vi "main.vi"() -> ()   [LabVIEW 2010]
uses:
  <vilib>/Platform/TimedLoop/XDataNode/wakeup.ctl
  <vilib>/Platform/TimedLoop/XDataNode/XDNodeRunTimeDep.lvlib
  <vilib>/Platform/TimedLoop/XDataNode/nitl_modes.ctl
  <vilib>/Platform/TimedLoop/XDataNode/timing_clust.ctl
  <vilib>/Platform/TimedLoop/XDataNode/XDataNode.xnode
  <vilib>/rvi/DataTransferAndStorage/Container/XNode/niFpgaContainer.xnode
  <vilib>/eio/EIONode/EIONode.xnode
  FPGA VIs/counter_cluster_flexRIO.ctl
  FPGA VIs/integration_cluster_flexRIO.ctl
  <vilib>/rvi/eio/nirviEIOImplementation/nirviEIOImplementation.xnode
  <vilib>/rvi/eio/common/nirviEmuTemplateMethod_noerrors.vi
  <vilib>/rvi/eio/common/nirviEmuClasses.ctl
  <vilib>/rvi/FIFO/Fifo_Resource/nirvififoEmulationSetSize.vi
  <vilib>/rvi/DataTransferAndStorage/Container/Common/niFpgaContainerGetUniqueNameForEmu.vi
  FPGA VIs/OnBoardBuffer_flexRIO Folder/OnBoardBuffer_flexRIO.lvlib
  FPGA VIs/OnBoardBuffer_flexRIO Folder/OnBoardBuffer_flexRIO.ctl
  common_typedefs/gate_parameters_cluster.ctl
  FPGA VIs/scan_specification_cluster_flexRIO.ctl
  FPGA VIs/derived_values_cluster_flexRIO.ctl
  FPGA VIs/DAC_voltage_cluster_flexRIO.ctl
  FPGA VIs/channels_cluster_flexRIO.ctl
  FPGA VIs/write_to_fifo_status_flexRIO.ctl
panel:
  out "read output":T1
  in  "channel offsets":T1
  out "derived values":T2
  out "integration loop counter":i32
  out "transferred z/intensity tuples":u32
  out "no of correct transferred z tuples":u32
  out "z-points transfer corrupt?":bool
  in  "transfer z-points?":bool
  out "transferred extra waitlines":u32
  in  "transfer extra-waitlines?":bool
  out "counter cluster out":T3
  out "pixels acquired":u64
  in  "scan":bool
  in  "wait for trigger?":bool
  in  "stop acquisition at\nFIFO overflow?":bool
  out "scanning?":bool
  out "loop-to-loop FIFO overflow":bool
  in  "stop":bool
  in  "scan specification":T4={"x amplitude"=1000, "x resolution (pixels)"=200, "x offset fly-forward (iterations)"=0, "x offset fly-back (iterations)"=0, "y resolution (nr. of lines)"=200, "y step size"=5, "iterations per pixel"=5, "number of frames"=-1, "y offset (pixels)"=0, "number of y-brake lines  (before y-fly-back)"=2, "number y-brake lines (after y-fly-back)"=2, "number of y-fly-back steps"=2, "lines per z step"=0, "number of z/intensity tuples"=0, "number of repetitions (volumes or planes)"=0}
  out "DAC voltages":T5 {"ch6" max=4095 step=1; "ch5" max=4095 step=1; "ch4" max=4095 step=1; "ch3" max=4095 step=1; "ch2" max=4095 step=1; "ch1" max=4095 step=1; "ch0" max=4095 step=1}
  out "acquire?":bool
  in  "sync minimum high":i16=1000
  in  "maximum bit depth":i8
  in  "enable fly-back reversion?":bool=TRUE
  in  "invert channels":bool[](array[boolean])=[FALSE, FALSE]
  out "no. elements in on-board buffer":u32
  out "on-board buffer":T6
  out "target-to-host FIFO full?":bool
  out "write-to-FIFO status":T7
  out "data received for buffering":u32
  in  "clock 1":T8
  in  "clock 2":T8
  in  "clock 3":T8
  out "clock 2 state":bool
  out "clock 1 state":bool
  out "clock 3 state":bool
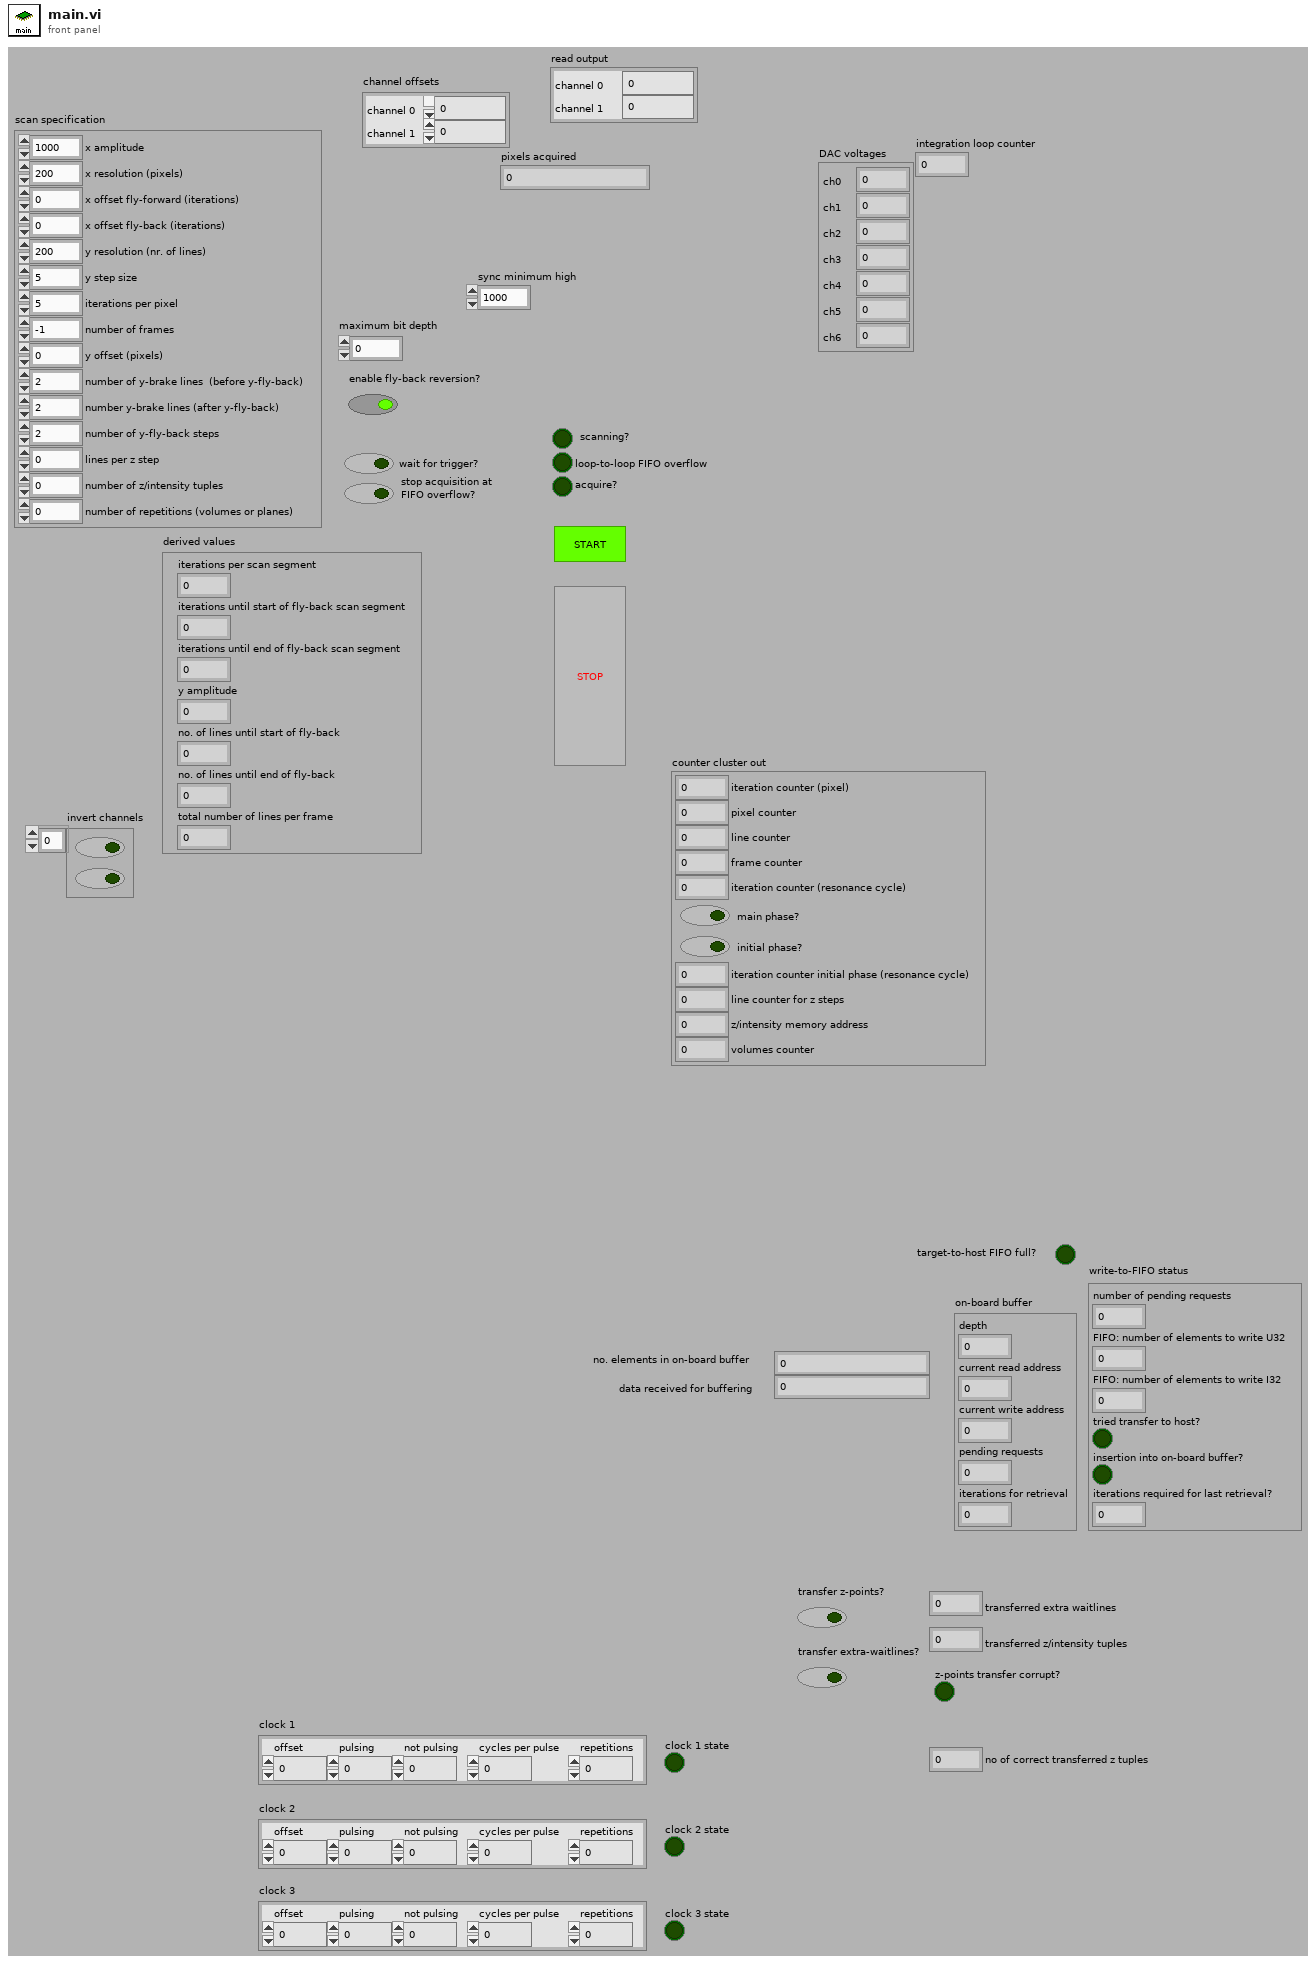
[diagram p1: front panel]
types:
  T1 = typedef "channels_cluster_flexRIO.ctl" = cluster{"channel 0":u32, "channel 1":u32}
  T2 = typedef "derived_values_cluster_flexRIO.ctl" = cluster{"iterations per scan segment":u16, "iterations until start of fly-back scan segment":u16, "iterations until end of fly-back scan segment":u16, "y amplitude":u16, "no. of lines until start of fly-back":u16, "no. of lines until end of fly-back":u16, "total number of lines per frame ":u16}
  T3 = typedef "counter_cluster_flexRIO.ctl" = cluster{"iteration counter (pixel)":u16, "pixel counter":u16, "line counter":u16, "frame counter":u16, "iteration counter (resonance cycle)":u16, "main phase?":bool, "initial phase?":bool, "iteration counter initial phase (resonance cycle)":u16, "line counter for z steps":u16, "z/intensity memory address":u32, "volumes counter":u16}
  T4 = typedef "scan_specification_cluster_flexRIO.ctl" = cluster{"x amplitude":u16, "x resolution (pixels)":u16, "x offset fly-forward (iterations)":u16, "x offset fly-back (iterations)":u16, "y resolution (nr. of lines)":u16, "y step size":u16, "iterations per pixel":u16, "number of frames":i32, "y offset (pixels)":u16, "number of y-brake lines  (before y-fly-back)":u16, "number y-brake lines (after y-fly-back)":u16, "number of y-fly-back steps":u16, "lines per z step":u16, "number of z/intensity tuples":u16, "number of repetitions (volumes or planes)":i32}
  T5 = typedef "DAC_voltage_cluster_flexRIO.ctl" = cluster{"ch0":u16, "ch1":u16, "ch2":u16, "ch3":u16, "ch4":u16, "ch5":u16, "ch6":u16}
  T6 = typedef "OnBoardBuffer_flexRIO.lvlib/OnBoardBuffer_flexRIO.ctl" = cluster{"depth":u32, "current read address":u32, "current write address":u32, "pending requests":u32, "iterations for retrieval":u32}
  T7 = typedef "write_to_fifo_status_flexRIO.ctl" = cluster{"number of pending requests":i32, "FIFO: number of elements to write U32":u32, "FIFO: number of elements to write I32":i32, "tried transfer to host?":bool, "insertion into on-board buffer?":bool, "iterations required for last retrieval?":u32}
  T8 = typedef "gate_parameters_cluster.ctl" = cluster{"offset":i64, "pulsing":i64, "not pulsing":i64, "cycles per pulse":i64, "repetitions":i64}
  T9 = typedef "integration_cluster_flexRIO.ctl" = cluster{"channel 0":u32, "channel 1":u32, "fly-back heap address":u32}
  T10 = typedef "XDNodeRunTimeDep.lvlib/timing_clust.ctl" = cluster{"Expected End [f-1]":u64, "Actual End [f-1]":u64, "Finished Late? [f-1]":bool, "Expected End [i-1]":u64, "Actual End [i-1]":u64, "Finished Late? [i-1]":bool, "Expected Start [i]":u64, "Actual Start [i]":u64, "Expected Start [f]":u64, "Actual Start [f]":u64, "Source Name":string, "Structure Name":string, "Period":i64, "Deadline":i64, "Offset":i64, "Start":i64, "Priority":i32, "Timeout":i32, "Mode":T11, "Wakeup Reason":T12, "Error":errorcluster, "Source Type":string, "Secondary Source Type":string, "Global End Time":u64, "Global Start Time":u64, "Frame Duration":u64, "Iteration Duration":u64, "Assigned CPU":i32, "I/O Scan Engine Mode":u32}
  T11 = typedef "XDNodeRunTimeDep.lvlib/nitl_modes.ctl" = enum32{"No Change", "Process missed periods, maintain original phase", "Discard missed periods, maintain original phase", "Process missed periods, ignore original phase", "Discard missed periods, ignore original phase"}
  T12 = typedef "XDNodeRunTimeDep.lvlib/wakeup.ctl" = enum32{"Normal", "Aborted", "Asynchronous wakeup", "Timing source error", "Timed loop error", "Timeout"}
  T13 = typedef "nirviEmuClasses.ctl" = enum16{"IO Read", "IO Write", "Method", "Property Read", "Property Write"}
  T14 = typedef "gate_counters_cluster.ctl" = cluster{"phase iteration counter":i64, "phase repetition counter":i64, "pulse iteration counter":i64, "phase state":bool}
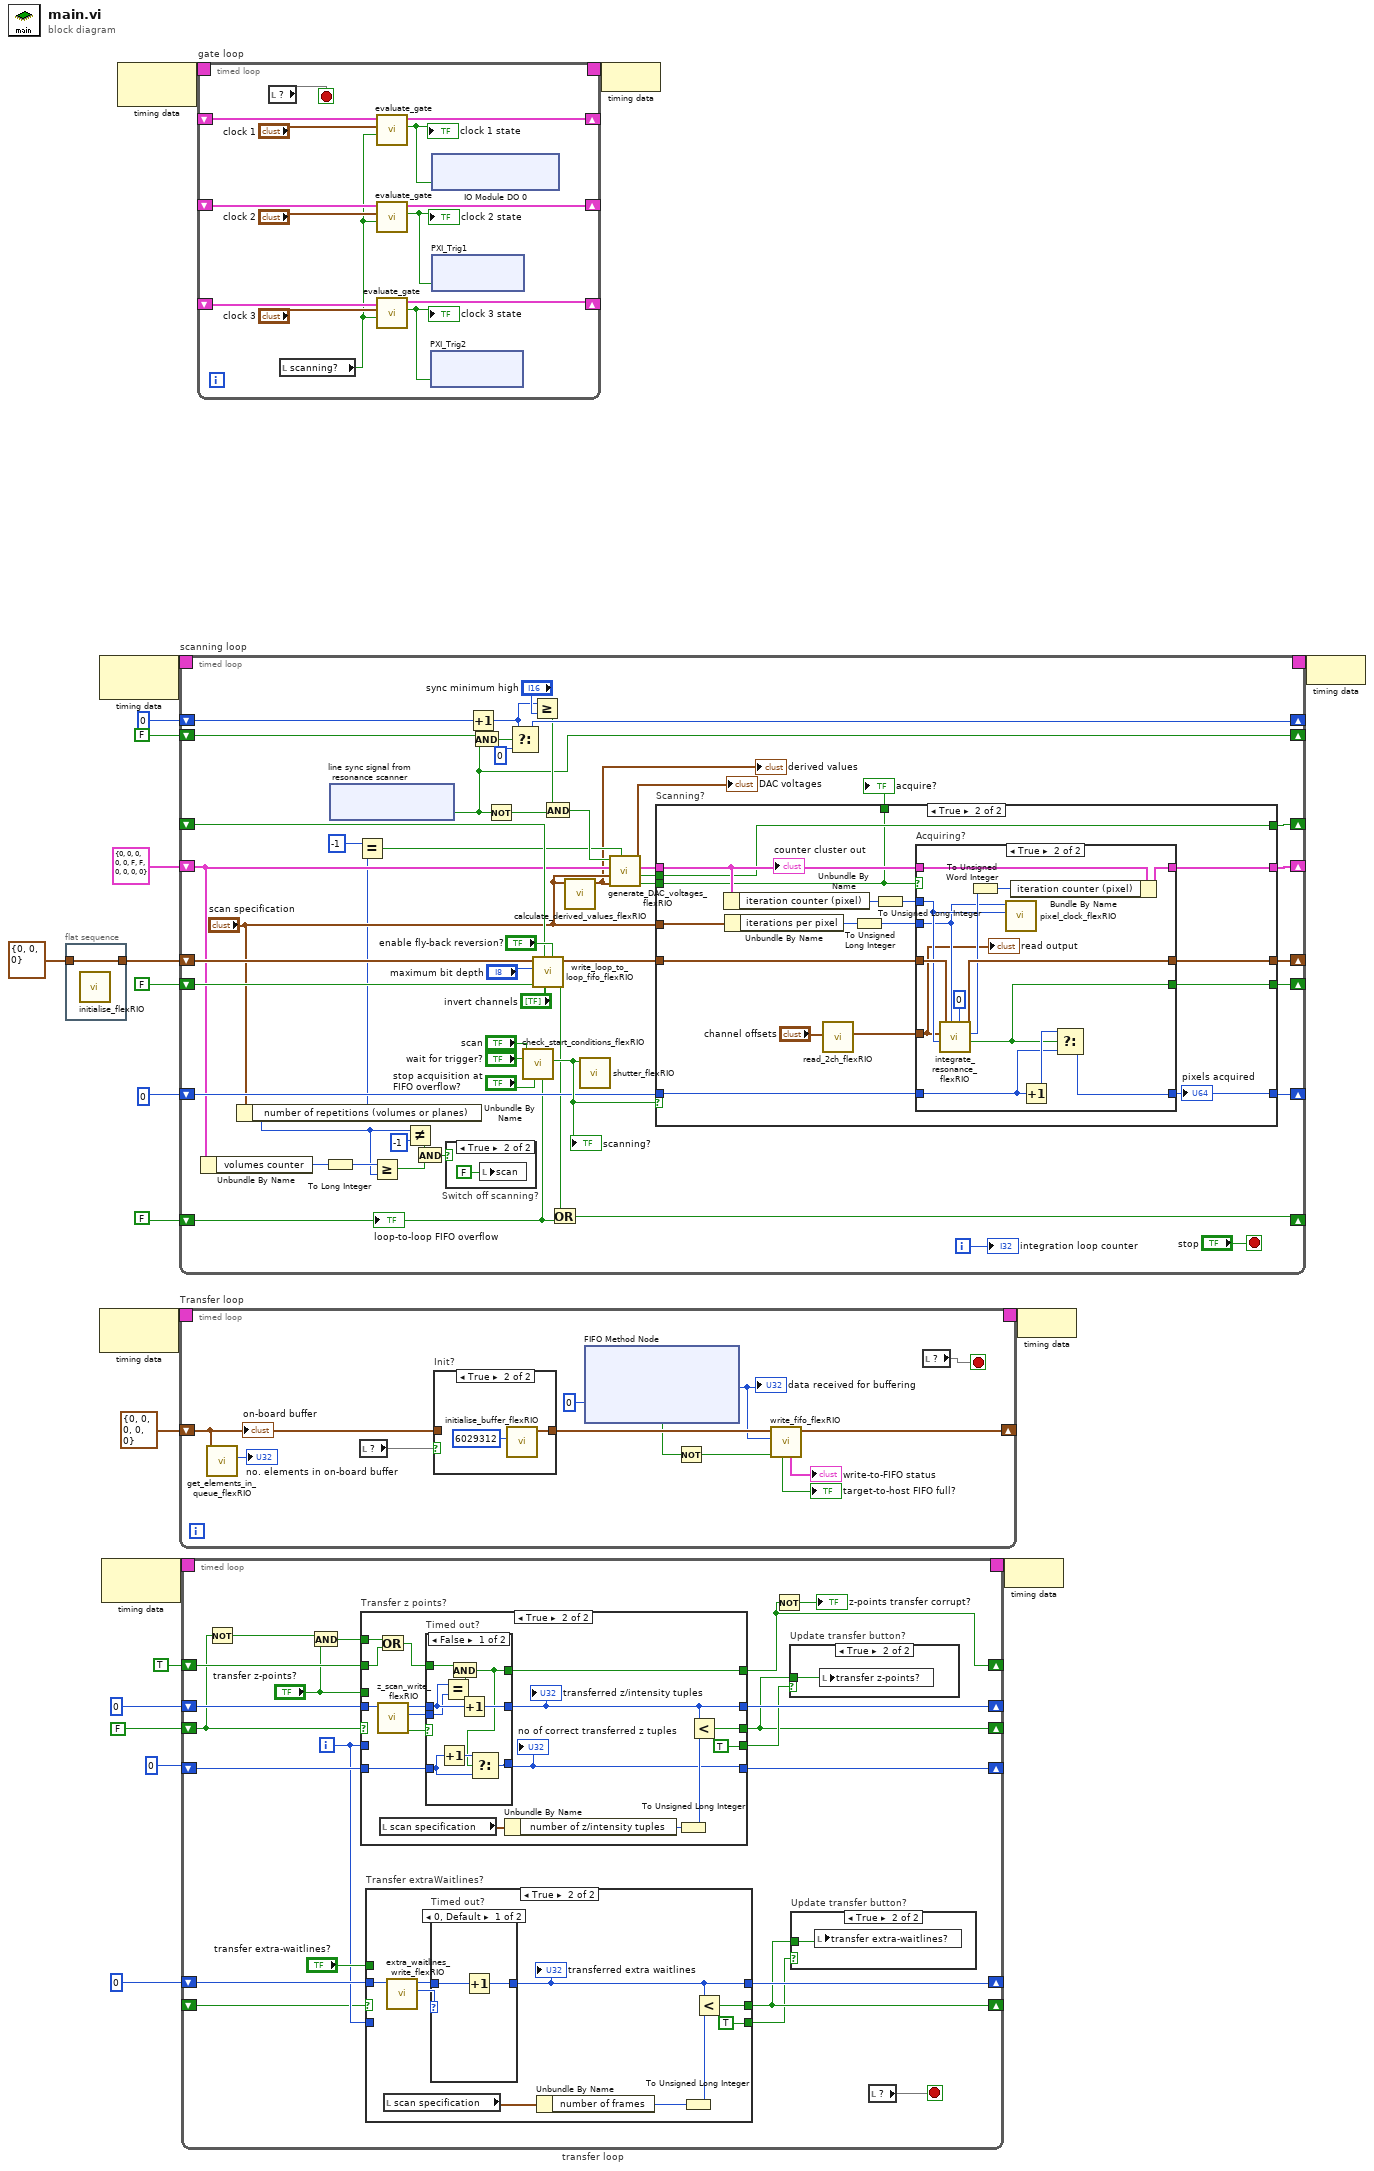
[diagram p0: block diagram]
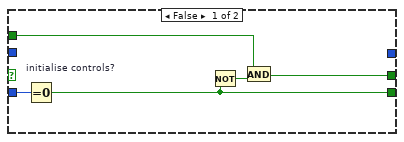
[diagram p3: hidden frame]
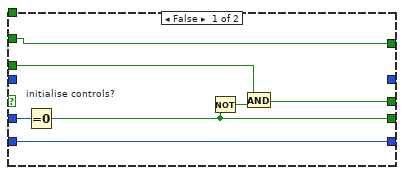
[diagram p6: hidden frame]
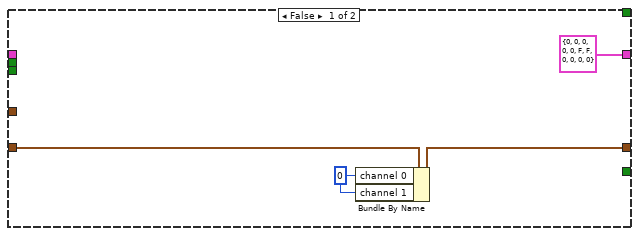
[diagram p9: hidden frame]
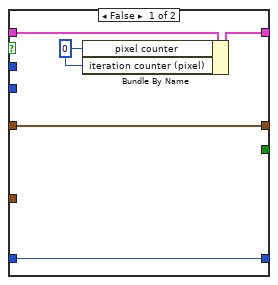
[diagram p10: hidden frame]
diagram:
  n1 = flat-sequence {
    tunnel: T9 {"channel 0"=0, "channel 1"=0, "fly-back heap address"=0} ("integration cluster") -> [w23]
    tunnel: [w23] -> w2
    frame #0 {
      n2 = call "initialise_flexRIO.vi"() -> ()  [unwired: 12 in]
    }
  }
  n3 = node-c288() -> (w18:T10)  [unwired: 1 in]
  n4 = node-c288() -> (w20:T10)  [unwired: 1 in]
  n5 = node-c288() -> (w10:T10)  [unwired: 1 in]
  n6 = node-c288() -> (w22:T10)  [unwired: 1 in]
  n7 = timed-loop "scanning loop" {
    timing: w18 -> [_]
    timing-out: [_] -> w17
    shift-right: [w71] -> _
    shift-left: T3 {"iteration counter (pixel)"=0, "pixel counter"=0, "line counter"=0, "frame counter"=0, "iteration counter (resonance cycle)"=0, "main phase?"=FALSE, "initial phase?"=FALSE, "iteration counter initial phase (resonance cycle)"=0, "line counter for z steps"=0, "z/intensity memory address"=0, "volumes counter"=0} ("counter cluster") -> [w37]
    shift-right: [w48] -> _
    shift-left: w2 -> [w47]
    shift-right: [w26] -> _
    shift-left: FALSE -> [w41]
    shift-right: [w40] -> _
    shift-left: FALSE -> [w60]
    shift-right: [w62] -> _
    shift-left: u64 0 -> [w63]
    shift-right: [w56] -> _
    shift-left: i16 0 -> [w59]
    shift-right: [w49] -> _
    shift-left: _ -> [w45]
    shift-right: [w43] -> _
    shift-left: FALSE ("finished?") -> [w42]
    i -> [w25]
    stop <- "stop" stop-if-true
    n8 = Unbundle By Name(w37) -> ("volumes counter"=w31:u16)
    n9 = Unbundle By Name("scan specification") -> ("number of repetitions (volumes or planes)"=w29:i32)
    n10 = To Long Integer(number=w31) -> (32bit integer=w30:i32)
    n11 = xnode "line sync signal from\nresonance scanner"() -> ("IO Module\\DI 1"=w40:bool)  [unwired: 1 in, 1 out]
    n12 = Equal?(x=-1, y=w29) -> (x = y?=w27:bool)
    n13 = Greater Or Equal?(x=w30, y=w29) -> (x >= y?=w68:bool)
    n14 = Not Equal?(x=w29, y=-1) -> (x != y?=w65:bool)
    n15 = And(x=w65, y=w68) -> (x .and. y?=w64:bool)
    n16 = case "Switch off scanning?" shown="True" w64 {
      frame False {
      }
      frame True {
        n17 = local write "scan"(FALSE ("scan")) -> ()
      }
    }
    n18 = Increment(x=w59) -> (x+1=w54:i16)
    n19 = And(x=w60, y=w40) -> (x .and. y?=w58:bool)
    n20 = Not(x=w40) -> (.not. x?=w53:bool)
    n21 = Select(t=w54, s=w58, f=i16 0) -> (s? t:f=w56:i16)
    n22 = call "check_start_conditions_flexRIO.vi"("FIFO overflow?"=w41, "stop at FIFO overflow?"="stop acquisition at\nFIFO overflow?", "in triggered mode?"="wait for trigger?", "acquire"="scan") -> ("acquire?"=w66:bool)  [unwired: 7 in]
    "scanning?" <- w66
    n23 = Greater Or Equal?(x=w54, y="sync minimum high") -> (x >= y?=w52:bool)
    n24 = call "write_loop_to_loop_fifo_flexRIO.vi"("enable fly-back reversion?"="enable fly-back reversion?", "invert channels"="invert channels", "fly-back?"=w45, "pixel finished?"=w42, "maximum bit depth"="maximum bit depth", "integration cluster in"=w47) -> ("local transfer FIFO full"=w44:bool, "integration cluster out"=w46:T9)  [unwired: 4 in]
    n25 = And(x=w52, y=w53) -> (x .and. y?=w38:bool)
    n26 = Or(x=w44, y=w41) -> (x .or. y?=w26:bool)
    n27 = call "calculate_derived_values_flexRIO.vi"("scan specification"="scan specification") -> ("derived values"=w24:T2)  [unwired: 10 in]
    "derived values" <- w24
    n28 = call "shutter_flexRIO.vi"("open?"=w66) -> ()  [unwired: 11 in]
    n29 = call "generate_DAC_voltages_flexRIO.vi"("focus mode?"=w27, "derived values"=w24, "scan specification"="scan specification", "counter cluster in"=w37, "resonant trigger"=w38) -> ("acquire?"=w33:bool, "fly-back acquisition phase?"=w34:bool, "counter cluster out"=w36:T3, "DAC voltages"=→"DAC voltages":T5)  [unwired: 3 in]
    n30 = case "Scanning?" shown="True" w66 {
      tunnel: w36 -> [_ w101]
      tunnel: [T3 {"iteration counter (pixel)"=0, "pixel counter"=0, "line counter"=0, "frame counter"=0, "iteration counter (resonance cycle)"=0, "main phase?"=FALSE, "initial phase?"=FALSE, "iteration counter initial phase (resonance cycle)"=0, "line counter for z steps"=0, "z/intensity memory address"=0, "volumes counter"=0} ("counter cluster") w113] -> w71
      tunnel: w46 -> [w95 w109]
      tunnel: [w94 w112] -> w48
      tunnel: "scan specification" -> [_ w102]
      tunnel: w63 -> [_ w105]
      tunnel: [_ w104] -> w62
      tunnel: [_ w99] -> w61
      tunnel: [_ w103] -> w43
      tunnel: [_ w100] -> w49
      tunnel: w34 -> [_ w100]
      tunnel: w33 -> [_ w99]
      frame False {
        w96 = u32 0 ("channel 0")
        n31 = Bundle By Name(cluster=w95, "channel 0"=w96, "channel 1"=w96) -> (w94:T9)
      }
      frame True {
        n32 = Unbundle By Name(w101) -> ("iteration counter (pixel)"=w111:u16)
        n33 = Unbundle By Name(w102) -> ("iterations per pixel"=w110:u16)
        n34 = call "read_2ch_flexRIO.vi"("channel offsets"="channel offsets") -> ("read output"=w107:T1)  [unwired: 10 in]
        n35 = To Unsigned Long Integer(number=w110) -> (unsigned 32bit integer=w106:u32)
        n36 = To Unsigned Long Integer(number=w111) -> (unsigned 32bit integer=w108:u32)
        n37 = case "Acquiring?" shown="True" w99 {
          tunnel: w101 -> [w117 w129]
          tunnel: [w118 w128] -> w113
          tunnel: [w114 w131] -> w112
          tunnel: w109 -> [w114 w126]
          tunnel: w108 -> [_ w121]
          tunnel: w107 -> [_ w119]
          tunnel: w106 -> [_ w120]
          tunnel: w105 -> [w116 w123]
          tunnel: [w116 w125] -> w104
          tunnel: [_ w122] -> w103
          frame False {
            w115 = u16 0 ("pixel counter")
            n38 = Bundle By Name(cluster=w117, "pixel counter"=w115, "iteration counter (pixel)"=w115) -> (w118:T3)
          }
          frame True {
            n39 = call "integrate_resonance_flexRIO.vi"("waiting iterations per pixel"=u32 0, "integration iterations per pixel"=w120, "iteration counter in"=w121, "sampling values in"=w119, "integration cluster in"=w126) -> ("finished?"=w122:bool, "iteration counter out"=w130:u32, "integration cluster out"=w131:T9)  [unwired: 4 in]
            n40 = To Unsigned Word Integer(number=w130) -> (unsigned 16bit integer=w132:u16)
            n41 = call "pixel_clock_flexRIO.vi"("current iteration"=w121, "iterations per pixel"=w120) -> ()  [unwired: 10 in]
            n42 = Bundle By Name(cluster=w129, "iteration counter (pixel)"=w132) -> (w128:T3)
            n43 = Increment(x=w123) -> (x+1=w124:u64)
            n44 = Select(t=w124, s=w122, f=w123) -> (s? t:f=w125:u64)
            "read output" <- w119
          }
        }
        "pixels acquired" <- w104
        "counter cluster out" <- w101
      }
    }
    "acquire?" <- w61
    "loop-to-loop FIFO overflow" <- w41
    "integration loop counter" <- w25
  }
  n45 = timed-loop "Transfer loop" {
    shift-right: [w142] -> _
    shift-left: T6 {"depth"=0, "current read address"=0, "current write address"=0, "pending requests"=0, "iterations for retrieval"=0} ("on-board buffer out") -> [w145]
    timing: w20 -> [_]
    timing-out: [_] -> w19
    stop <- w140 stop-if-true
    n46 = call "get_elements_in_queue_flexRIO.vi"("on-board buffer in"=w145) -> ("no. elements"=→"no. elements in on-board buffer":u32)  [unwired: 10 in]
    n47 = local read item#-1() -> (w144)
    n48 = case "Init?" shown="True" w144 {
      tunnel: [w198 w200] -> w143
      tunnel: w145 -> [w198 _]
      frame False {
      }
      frame True {
        n49 = call "initialise_buffer_flexRIO.vi"("depth"=u32 6029312) -> ("on-board buffer out"=w200:T6)  [unwired: 10 in]
      }
    }
    n50 = xnode ("FIFO Method Node")("Timeout"=0) -> ("Element"=w139:u32, "Timed Out?"=w136:bool)  [unwired: 1 in, 1 out]
    "data received for buffering" <- w139
    n51 = Not(x=w136) -> (.not. x?=w135:bool)
    n52 = call "write_fifo_flexRIO.vi"("input ready?"=w135, "data"=w139, "on-board buffer in"=w143) -> ("on-board buffer out"=w142:T6, "write-to-FIFO status"=→"write-to-FIFO status":T7, "FIFO full?"=→"target-to-host FIFO full?":bool)  [unwired: 6 in]
    n53 = local read item#-1() -> (w140)
    "on-board buffer" <- w145
  }
  n54 = timed-loop "transfer loop" {
    shift-right: [w222] -> _
    shift-left: u32 0 ("address out") -> [w223]
    timing: w10 -> [_]
    timing-out: [_] -> w9
    shift-right: [w219] -> _
    shift-left: FALSE ("start z-points transfer?") -> [w214]
    shift-right: [w217] -> _
    shift-left: TRUE ("start z-points transfer?") -> [w218]
    shift-right: [w210] -> _
    shift-left: u32 0 ("address out") -> [w211]
    shift-right: [w208] -> _
    shift-left: u32 0 ("address extra waitlines OUT") -> [w209]
    shift-right: [w204] -> _
    shift-left: _ -> [w205]
    i -> [w206]
    stop <- w221 stop-if-true
    n55 = Not(x=w214) -> (.not. x?=w215:bool)
    n56 = And(x=w215, y="transfer z-points?") -> (x .and. y?=w212:bool)
    n57 = case "Transfer z points?" shown="True" w214 {
      tunnel: w223 -> [_ w265]
      tunnel: [_ w263] -> w222
      tunnel: [w247 w259] -> w219
      tunnel: w206 -> [w249 _]
      tunnel: [w246 TRUE] -> w220
      tunnel: w218 -> [w245 w253]
      tunnel: [w245 w255] -> w217
      tunnel: "transfer z-points?" -> [w244 _]
      tunnel: w212 -> [_ w254]
      tunnel: w211 -> [w243 w251]
      tunnel: [w243 w250] -> w210
      frame False {
        n58 = Equal To 0? "initialise controls?"(x=w249) -> (x = 0?=w246:bool)
        n59 = Not(x=w246) -> (.not. x?=w248:bool)
        n60 = And(x=w244, y=w248) -> (x .and. y?=w247:bool)
      }
      frame True {
        n61 = Or(x=w254, y=w253) -> (x .or. y?=w252:bool)
        n62 = call "z_scan_write_flexRIO.vi"("address in"=w265) -> ("FIFO scan time out"=w257:bool, "data"=w256:u32, "address out"=w264:u32)  [unwired: 8 in]
        n63 = local read "scan specification"() -> (w262:T4)
        n64 = case "Timed out?" shown="False" w257 {
          tunnel: w264 -> [w271 w277]
          tunnel: [w274 w277] -> w263
          tunnel: w256 -> [w270 _]
          tunnel: w252 -> [w273 w276]
          tunnel: [w267 w276] -> w255
          tunnel: w251 -> [w269 w275]
          tunnel: [w266 w275] -> w250
          frame False {
            n65 = Increment(x=w269) -> (x+1=w268:u32)
            n66 = Equal?(x=w271, y=w270) -> (x = y?=w272:bool)
            n67 = And(x=w273, y=w272) -> (x .and. y?=w267:bool)
            n68 = Increment(x=w271) -> (x+1=w274:u32)
            n69 = Select(t=w268, s=w267, f=w269) -> (s? t:f=w266:u32)
          }
          frame True {
          }
        }
        "transferred z/intensity tuples" <- w263
        "no of correct transferred z tuples" <- w250
        n70 = Unbundle By Name(w262) -> ("number of z/intensity tuples"=w261:u16)
        n71 = To Unsigned Long Integer(number=w261) -> (unsigned 32bit integer=w260:u32)
        n72 = Less?(x=w263, y=w260) -> (x < y?=w259:bool)
      }
    }
    n73 = case "Transfer extraWaitlines?" shown="True" w205 {
      tunnel: [_ w238] -> w208
      tunnel: [w228 w235] -> w204
      tunnel: [w227 TRUE] -> w203
      tunnel: w209 -> [_ w231]
      tunnel: "transfer extra-waitlines?" -> [w225 _]
      tunnel: w206 -> [w226 _]
      frame False {
        n74 = Equal To 0? "initialise controls?"(x=w226) -> (x = 0?=w227:bool)
        n75 = Not(x=w227) -> (.not. x?=w229:bool)
        n76 = And(x=w225, y=w229) -> (x .and. y?=w228:bool)
      }
      frame True {
        n77 = local read "scan specification"() -> (w233:T4)
        n78 = call "extra_waitlines_write_flexRIO.vi"("address extra waitlines IN"=w231) -> ("data"=w230:u32, "address extra waitlines OUT"=w232:u32)  [unwired: 8 in, 1 out]
        n79 = case "Timed out?" shown="0, Default" w230 {
          tunnel: w232 -> [w239 w241]
          tunnel: [w240 w241] -> w238
          frame 0, Default {
            n80 = Increment(x=w239) -> (x+1=w240:u32)
          }
          frame 1 {
          }
        }
        "transferred extra waitlines" <- w238
        n81 = Unbundle By Name(w233) -> ("number of frames"=w237:i32)
        n82 = To Unsigned Long Integer(number=w237) -> (unsigned 32bit integer=w236:u32)
        n83 = Less?(x=w238, y=w236) -> (x < y?=w235:bool)
      }
    }
    n84 = Not(x=w217) -> (.not. x?=→"z-points transfer corrupt?":bool)
    n85 = case "Update transfer button?" shown="True" w220 {
      tunnel: w219 -> [_ w242]
      frame False {
      }
      frame True {
        n86 = local write "transfer z-points?"(w242) -> ()
      }
    }
    n87 = case "Update transfer button?" shown="True" w203 {
      tunnel: w204 -> [_ w224]
      frame False {
      }
      frame True {
        n88 = local write "transfer extra-waitlines?"(w224) -> ()
      }
    }
    n89 = local read item#-1() -> (w221)
  }
  n90 = timed-loop "gate loop" {
    timing: w22 -> [_]
    timing-out: [_] -> w21
    shift-right: [w292] -> _
    shift-left: _ -> [w293]
    shift-right: [w290] -> _
    shift-left: _ -> [w291]
    shift-right: [w289] -> _
    shift-left: _ -> [w288]
    stop <- w285 stop-if-true
    n91 = local read item#-1() -> (w285)
    n92 = local read "scanning?"() -> (w280:bool)
    n93 = call "evaluate_gate.vi"("acquiring?"=w280, "gate settings"="clock 1", "gate counters in"=w293) -> ("pulse state out"=w282:bool, "gate counters out"=w292:T14)  [unwired: 7 in]
    "clock 1 state" <- w282
    n94 = call "evaluate_gate.vi"("acquiring?"=w280, "gate settings"="clock 2", "gate counters in"=w291) -> ("pulse state out"=w284:bool, "gate counters out"=w290:T14)  [unwired: 7 in]
    "clock 2 state" <- w284
    n95 = call "evaluate_gate.vi"("acquiring?"=w280, "gate settings"="clock 3", "gate counters in"=w288) -> ("pulse state out"=w283:bool, "gate counters out"=w289:T14)  [unwired: 7 in]
    "clock 3 state" <- w283
    n96 = xnode "PXI_Trig2"("PXI_Trig2"=w283) -> ()  [unwired: 1 in, 1 out]
    n97 = xnode "IO Module DO 0"("IO Module\\D0 0"=w282) -> ()  [unwired: 1 in, 1 out]
    n98 = xnode "PXI_Trig1"("PXI_Trig1"=w284) -> ()  [unwired: 1 in, 1 out]
  }
  n99 = node-c288(w21) -> ()
  n100 = node-c288(w9) -> ()
  n101 = node-c288(w19) -> ()
  n102 = node-c288(w17) -> ()
